vi "3.0 - Functional Array Holding Global.vi"(1 "Input Act Neurons":T2, 2 "Mode":T1(ring)=enum."Read Joystick") -> (0 "Output Act Neurons":T2)   [LabVIEW 2011]
uses:
  4-High Neurons/4.1.2-Act Neuron TD.ctl
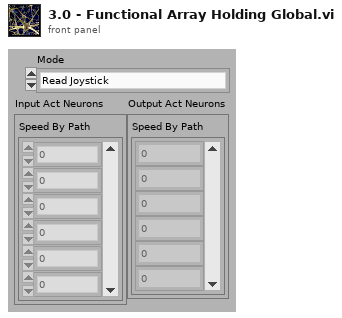
[diagram p1: front panel]
types:
  T1 = enum16{"Set Joystick", "Read Joystick", "Set Forebrain", "Read Forebrain", "Set Limbic", "Read Limbic", "Set Cerebellum", "Read Cerebellum", "Set Arbitrated", "Read Arbitrated", "Set LIDAR", "Read LIDAR", "Read Shallow Map", "Set Shallow Map", "Read Decider", "Set Decider"}
  T2 = typedef "4.1.2-Act Neuron TD.ctl" = cluster{"Speed By Path":sgl[]}
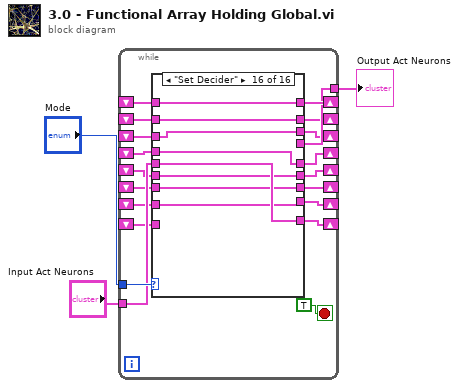
[diagram p0: block diagram]
diagram:
  n1 = while {
    shift-right: [w22] -> _
    shift-left: _ -> [w18]
    tunnel: "Mode" -> [w21]
    tunnel: "Input Act Neurons" -> [w20]
    tunnel: [w19] -> w1
    shift-right: [w17] -> _
    shift-left: _ -> [w16]
    shift-right: [w15] -> _
    shift-left: _ -> [w14]
    shift-right: [w13] -> _
    shift-left: _ -> [w12]
    shift-right: [w11] -> _
    shift-left: _ -> [w10]
    shift-right: [w9] -> _
    shift-left: _ -> [w8]
    shift-right: [w6] -> _
    shift-left: _ -> [w7]
    shift-right: [w5] -> _
    shift-left: _ -> [w4]
    stop <- TRUE stop-if-true
    n2 = case shown="\"Set Decider\"" w21 {
      tunnel: [w32 w40 w49 w57 w66 w74 w83 w91 w100 w108 w117 w125 w127 w135 w142 w156] -> w22
      tunnel: w20 -> [w32 _ w48 _ w64 _ w80 _ w96 _ w112 _ _ w141 _ w157]
      tunnel: [w31 w40 w47 w56 w63 w72 w79 w88 w95 w104 w111 w120 w132 _ w148 _] -> w19
      tunnel: w18 -> [w31 w40 w49 w57 w66 w74 w83 w91 w100 w108 w117 w125 w127 w135 w142 w156]
      tunnel: [w30 w39 w48 w56 w65 w73 w82 w90 w99 w107 w116 w124 w128 w137 w143 w155] -> w17
      tunnel: w16 -> [w30 w39 w47 w56 w65 w73 w82 w90 w99 w107 w116 w124 w128 w137 w143 w155]
      tunnel: [w29 w38 w46 w55 w64 w72 w81 w89 w98 w106 w115 w123 w129 w136 w144 w154] -> w15
      tunnel: w14 -> [w29 w38 w46 w55 w63 w72 w81 w89 w98 w106 w115 w123 w129 w136 w144 w154]
      tunnel: [w28 w37 w45 w54 w62 w71 w80 w88 w97 w105 w114 w122 w130 w138 w145 w153] -> w13
      tunnel: w12 -> [w28 w37 w45 w54 w62 w71 w79 w88 w97 w105 w114 w122 w130 w138 w145 w153]
      tunnel: [w27 w36 w44 w53 w61 w70 w78 w87 w96 w104 w113 w121 w131 w140 w146 w152] -> w11
      tunnel: w10 -> [w27 w36 w44 w53 w61 w70 w78 w87 w95 w104 w113 w121 w131 w140 w146 w152]
      tunnel: [w26 w35 w43 w52 w60 w69 w77 w86 w94 w103 w112 w120 w133 w139 w147 w151] -> w9
      tunnel: w8 -> [w26 w35 w43 w52 w60 w69 w77 w86 w94 w103 w111 w120 w133 w139 w147 w151]
      tunnel: w7 -> [w25 w34 w42 w51 w59 w68 w76 w85 w93 w102 w110 w119 w132 _ w149 w150]
      tunnel: [w25 w34 w42 w51 w59 w68 w76 w85 w93 w102 w110 w119 w132 w141 w149 w150] -> w6
      tunnel: [w24 w33 w41 w50 w58 w67 w75 w84 w92 w101 w109 w118 w126 w134 w148 w157] -> w5
      tunnel: w4 -> [w24 w33 w41 w50 w58 w67 w75 w84 w92 w101 w109 w118 w126 w134 w148 _]
      frame "Set Joystick", Default {
      }
      frame "Read Joystick" {
      }
      frame "Set Forebrain" {
      }
      frame "Read Forebrain" {
      }
      frame "Set Limbic" {
      }
      frame "Read Limbic" {
      }
      frame "Set Cerebellum" {
      }
      frame "Read Cerebellum" {
      }
      frame "Set Arbitrated" {
      }
      frame "Read Arbitrated" {
      }
      frame "Set LIDAR" {
      }
      frame "Read LIDAR" {
      }
      frame "Read Shallow Map" {
      }
      frame "Set Shallow Map" {
      }
      frame "Read Decider" {
      }
      frame "Set Decider" {
      }
    }
  }
  "Output Act Neurons" <- w1
